vi "Perform Action.vi"(8 "error in (no error)":errorcluster, 10 "Input":variant, 11 "Virtual Instrument in":refnum<class "Virt Voltage Reader.lvclass">) -> (0 "error out":errorcluster, 2 "Output":variant, 3 "Virtual Instrument out":refnum<class "Virt Voltage Reader.lvclass">)   [LabVIEW 2023, in "Scope Base.lvlib" / "Virt Voltage Reader.lvclass"]
uses:
  Virt Voltage Reader.lvclass
  Virtual Instrument Base/Virtual Instrument Base.lvclass
  Virt Voltage Reader.lvclass/Virt Voltage Reader.ctl
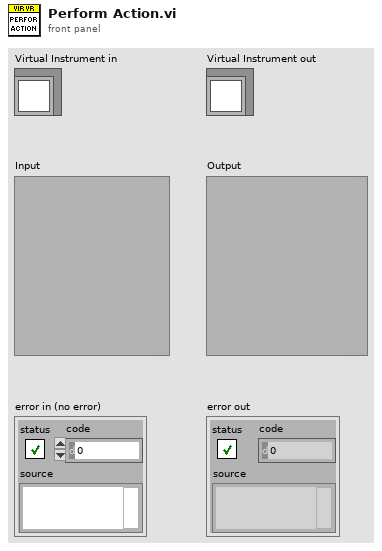
[diagram p1: front panel]
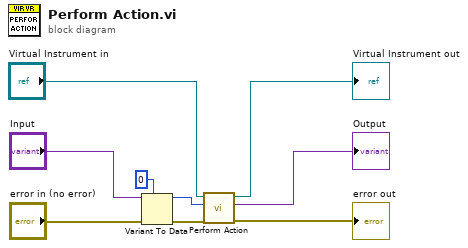
[diagram p0: block diagram]
diagram:
  n1 = Variant To Data(error in="error in (no error)", type=u8 0, Variant="Input") -> (data=w5:u8, error out=w6:errorcluster)
  n2 = call-parent "Perform Action.vi"("error in (no error)"=w6, "Input"=w5, "Virtual Instrument in"="Virtual Instrument in") -> ("error out"=→"error out":errorcluster, "Output"=→"Output":variant, "Virtual Instrument out"=→"Virtual Instrument out":refnum<class "Virt Voltage Reader.lvclass">)  [unwired: 6 in]
